vi "Save_Test.vi"() -> ()   [LabVIEW 2018]
panel:
  in  "element 14":dbl
  in  "Commentary":string
  in  "TuneFile":string
  in  "TEQComment":string
  in  "TEQFile":string
  in  "QComment":string
  in  "QCurveFile":string
  in  "Save_Path":string
  in  "Task3Pressure":dbl
  in  "Task3Temperature":dbl
  in  "NMRChannel":dbl
  in  "element 13":dbl
  in  "IfAtten":dbl
  in  "BeamON":dbl
  in  "RFLevel":dbl
  in  "Fupper":dbl
  in  "FLower":dbl
  in  "PeakCenter":dbl
  in  "PeakAmp":dbl
  out "return value":string
  in  "module path":path
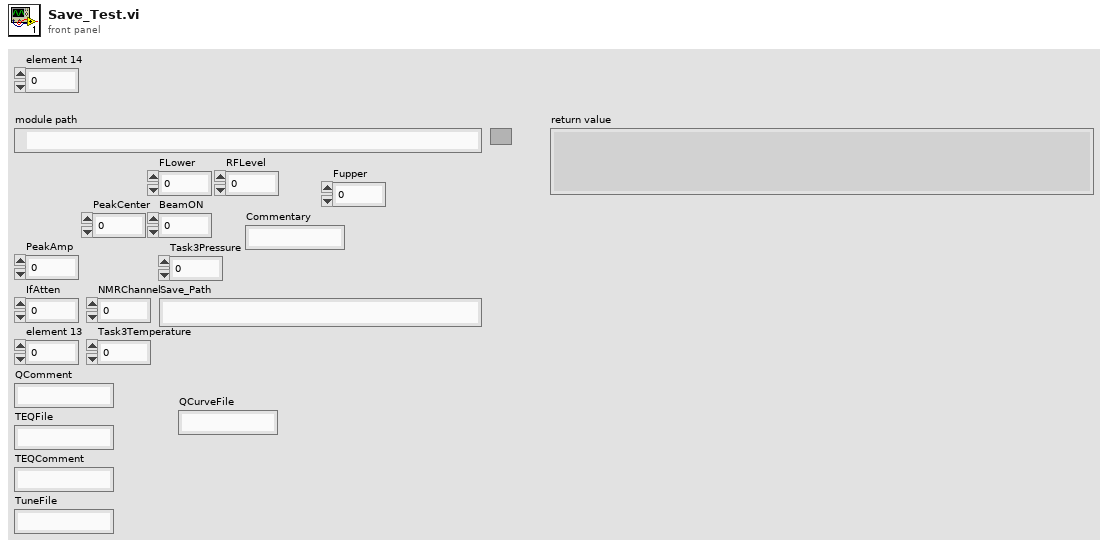
[diagram p1: front panel]
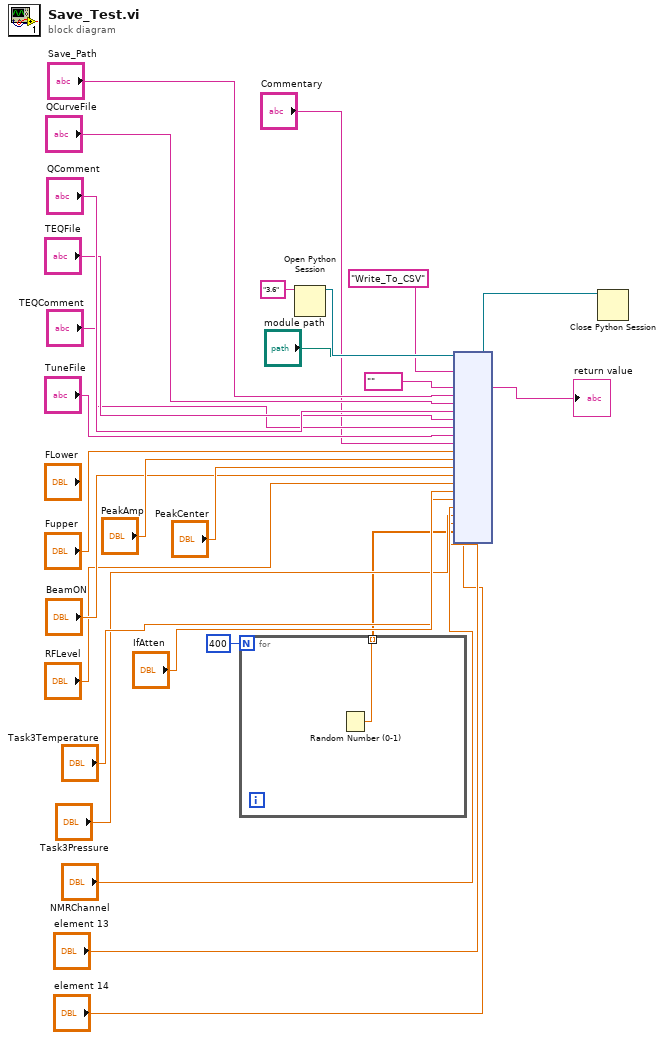
[diagram p0: block diagram]
diagram:
  n1 = for {
    N: 400 -> [_]
    tunnel: [w28] -> w2 mode=indexing
    n2 = Random Number (0-1)() -> (number: 0 to 1=w28:dbl)
  }
  n3 = Open Python Session(python version="3.6" ("Python version")) -> (session out=w27:refnum<k35>)  [unwired: 2 in, 1 out]
  n4 = node(w27, "module path", "Write_To_CSV" ("function name"), "", "Save_Path", "QCurveFile", "QComment", "TEQFile", "TEQComment", "TuneFile", "Commentary", "Fupper", "PeakAmp", "PeakCenter", "BeamON", "RFLevel", "IfAtten", "Task3Temperature", "NMRChannel", "Task3Pressure", "element 13", w2, "element 14") -> (w26:refnum<k35>, →"return value":string)  [unwired: 20 in, 3 out]
  n5 = Close Python Session(session in=w26) -> ()  [unwired: 1 in, 1 out]
